vi "oauth2_token_code.vi"(6 "redirect_uri":string, 8 "error in (no error)":errorcluster, 9 "client_secret":string, 10 "client_id":string, 11 "authorization_code":string) -> (0 "error out":errorcluster, 3 "access_token":string)   [LabVIEW 2015, in "lv-dropbox.lvlib"]
uses:
  lv-dropbox.lvlib
  private/_controls/content_type.ctl
  <vilib>/httpClient/POSTBuffer.vi
  <vilib>/httpClient/LabVIEWHTTPClient.lvlib
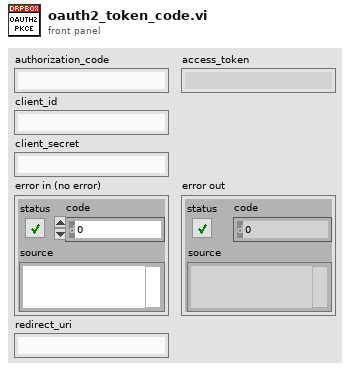
[diagram p1: front panel]
types:
  T1 = typedef "lv-dropbox.lvlib/content_type.ctl" = enum16{"<content_type>", "application/json", "application/octet-stream", "application/x-www-form-urlencoded"}
  T2 = cluster{"access_token":string, "expires_in":dbl, "token_type":string}
  T3 = typedef "LabVIEWHTTPClient.lvlib/ClientHandle.ctl" = refnum<k1>
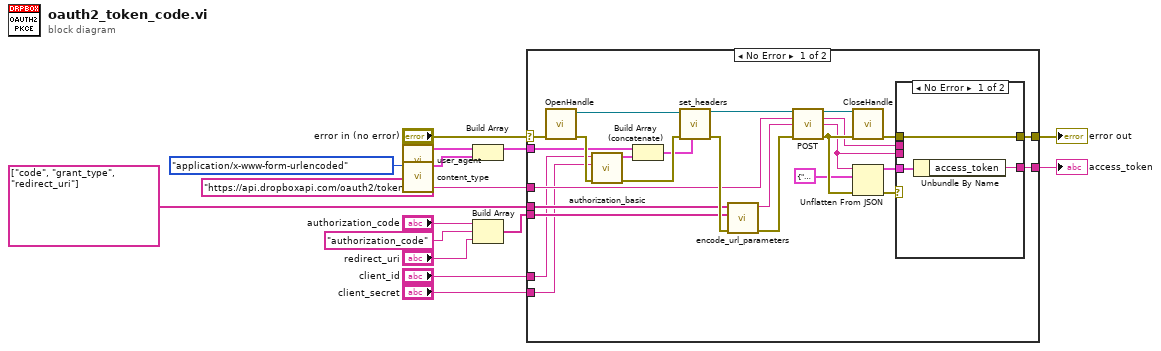
[diagram p0: block diagram]
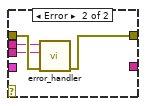
[diagram p2: hidden frame]
diagram:
  n1 = call "user_agent.vi"() -> ("header"=w12:cluster{"header":string, "value":string})  [unwired: 11 in]
  n2 = call "content_type.vi"("content_type"=content_type."application/x-www-form-urlencoded") -> ("header"=w14:cluster{"header":string, "value":string})  [unwired: 10 in]
  n3 = Build Array(w12, w14) -> (w11:cluster{"header":string, "value":string}[])
  n4 = Build Array("authorization_code", "authorization_code", "redirect_uri") -> (w6:string[])
  n5 = case shown="No Error" "error in (no error)" {
    selector: "error in (no error)" -> [w16 w49]
    tunnel: "https://api.dropboxapi.com/oauth2/token" ("url") -> [w37 _]
    tunnel: w11 -> [w33 _]
    tunnel: [w28 w49] -> w13
    tunnel: string[] ["code", "grant_type", "redirect_uri"] -> [w24 _]
    tunnel: [w25 _] -> w8
    tunnel: w6 -> [w23 _]
    tunnel: "client_id" -> [w18 _]
    tunnel: "client_secret" -> [w17 _]
    frame No Error {
      n6 = call <vilib>:"OpenHandle.vi"("error in (no error)"=w16) -> ("client handle out"=w34:T3, "error out"=w41:errorcluster)  [unwired: 13 in]
      n7 = call "authorization_basic.vi"("error in (no error)"=w41, "password"=w17, "username"=w18) -> ("error out"=w40:errorcluster, "header"=w19:cluster{"header":string, "value":string})  [unwired: 7 in]
      n8 = Build Array (concatenate)(w33, w19) -> (w20:cluster{"header":string, "value":string}[])
      n9 = call "set_headers.vi"("header_value []"=w20, "error in (no error)"=w40, "client_handle in"=w34) -> ("error out"=w39:errorcluster, "client_handle out"=w32:T3)  [unwired: 7 in]
      n10 = call "encode_url_parameters.vi"("error in (no error)"=w39, "value []"=w23, "key []"=w24) -> ("error out"=w21:errorcluster, "url_encoded_string"=w22:string)  [unwired: 7 in]
      n11 = call-poly <vilib>:"POST.vi"("client handle"=w32, "url"=w37, "buffer"=w22, "error in (no error)"=w21) -> ("client handle out"=w31:T3, "headers"=w27:string, "body"=w26:string, "error out"=w38:errorcluster)  [unwired: 8 in]
      n12 = call <vilib>:"CloseHandle.vi"("client handle"=w31, "error in (no error)"=w38) -> ("error out"=w29:errorcluster)  [unwired: 13 in]
      n13 = Unflatten From JSON(JSON string=w26, type and defaults=T2 {"access_token"="", "expires_in"=0.0, "token_type"=""} ("value"), error in (no error)=w38) -> (value=w35:T2, error out=w30:errorcluster)  [unwired: 4 in]
      n14 = case shown="No Error" w30 {
        tunnel: w35 -> [w43 _]
        tunnel: w29 -> [w44 w48]
        tunnel: [w44 w45] -> w28
        tunnel: w27 -> [_ w47]
        tunnel: w26 -> [_ w46]
        tunnel: [w42 _] -> w25
        frame No Error {
          n15 = Unbundle By Name(w43) -> ("access_token"=w42:string)
        }
        frame Error {
          n16 = call "error_handler.vi"("error in (no error)"=w48, "body"=w46, "headers"=w47) -> ("error out"=w45:errorcluster)  [unwired: 8 in]
        }
      }
    }
    frame Error {
    }
  }
  "error out" <- w13
  "access_token" <- w8
